vi "Unload.vi"(8 "error in":errorcluster, 11 "GrabberTool in":refnum<class "GrabberTool Class.lvclass">) -> (0 "error out":errorcluster, 3 "Gantry out":refnum<class "Gantry Class.lvclass">)   [LabVIEW 2011, in "GrabberTool Class.lvclass"]
uses:
  GrabberTool Class.lvclass
  Gantry Class/Gantry Class.lvclass
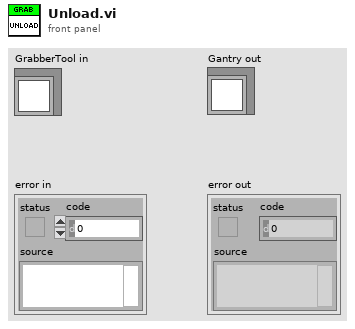
[diagram p1: front panel]
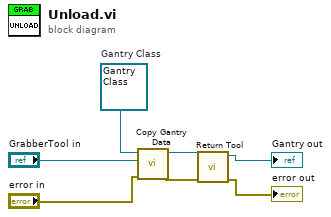
[diagram p0: block diagram]
diagram:
  w7 = refnum<class "Gantry Class.lvclass"> refnum  # Gantry Class
  n1 = call "Copy Gantry Data.vi"("error in"="error in", "Gantry Source"="GrabberTool in", "Gantry Dest"=w7) -> ("error out"=w2:errorcluster, "Gantry Result"=w4:refnum<class "Gantry Class.lvclass">)  [unwired: 7 in]
  n2 = call-dynamic "Return Tool.vi"("error in"=w2, "Gantry in"=w4) -> ("error out"=→"error out":errorcluster, "Gantry out"=→"Gantry out":refnum<class "Gantry Class.lvclass">)  [unwired: 8 in]
